vi "select time.vi"(8 "error in (no error)":errorcluster, 10 "N attemt=0":bool, 11 "MB_TCP in":refnum<class "MB_TCP.lvclass">) -> (0 "error out":errorcluster, 3 "MB_TCP out":refnum<class "MB_TCP.lvclass">)   [LabVIEW 2021, in "MB_TCP.lvclass"]
uses:
  MB_TCP.lvclass
  MB_TCP.lvclass/MB_TCP.ctl
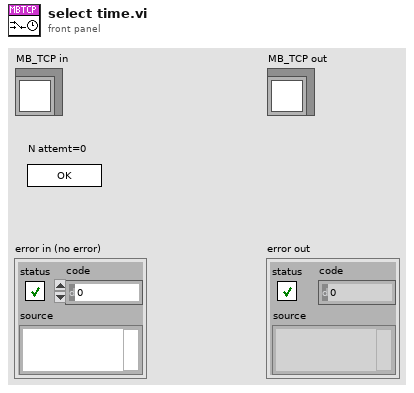
[diagram p1: front panel]
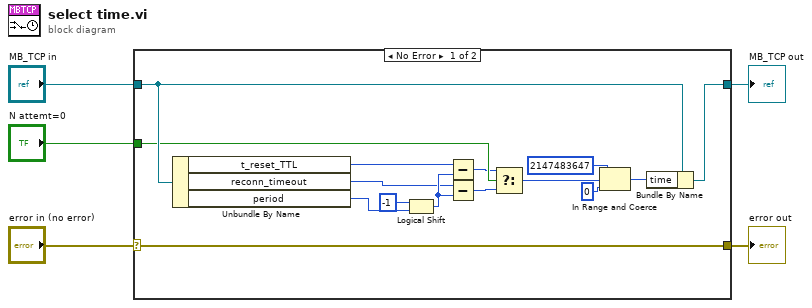
[diagram p0: block diagram]
diagram:
  n1 = case shown="No Error" "error in (no error)" {
    selector: "error in (no error)" -> [w20 w21]
    tunnel: [w20 w21] -> w4
    tunnel: [w19 w22] -> w2
    tunnel: "MB_TCP in" -> [w18 w22]
    tunnel: "N attemt=0" -> [w12 _]
    frame No Error {
      n2 = Unbundle By Name(w18) -> ("t_reset_TTL"=w15:i32, "reconn_timeout"=w14:i32, "period"=w13:i32)
      n3 = Logical Shift(y=i16 -1, x=w13) -> (x << y=w16:i32)
      n4 = Subtract(x=w15, y=w16) -> (x-y=w11:i32)
      n5 = Subtract(x=w14, y=w16) -> (x-y=w10:i32)
      n6 = Select(t=w11, s=w12, f=w10) -> (s? t:f=w9:i32)
      n7 = In Range and Coerce(upper limit=2147483647, x=w9, lower limit=0) -> (coerced(x)=w8:i32)  [unwired: 1 out]
      n8 = Bundle By Name(cluster=w18, "time"=w8) -> (w19:refnum<class "MB_TCP.lvclass">)
    }
    frame Error {
    }
  }
  "error out" <- w4
  "MB_TCP out" <- w2
